vi "Matrix Inverse v1.3.vi"() -> ()   [LabVIEW 2020]
uses:
  <vilib>/Analysis/Matrix/Datatypes/RealMatrix.ctl
  <vilib>/Analysis/baseanly.llb/Mean (DBL).vi
  <vilib>/Analysis/Matrix/Numeric/Conversions/Array To Matrix - RA2.vi
  <vilib>/Analysis/baseanly.llb/Real Inverse Matrix.vi
  <vilib>/Analysis/Matrix/Numeric/Conversions/Matrix To Array - RM.vi
  <vilib>/Analysis/NI_AALBase.lvlib
  <vilib>/Analysis/Matrix/NI_Matrix.lvlib
panel:
  out "pt - pt error":sgl[][](array[numeric])
  out "percent error":dbl format="%0.2f"
  out "x > y?":bool
  out "divide by zero detected":bool
  out "Joint Matrix":sgl[][](array[numeric])
  out "A":T1
  out "sum of error":sgl
  out "inv(A) LABVIEW-FPGA":sgl[][](array[numeric])
  out "inv(A) LABVIEW":T1
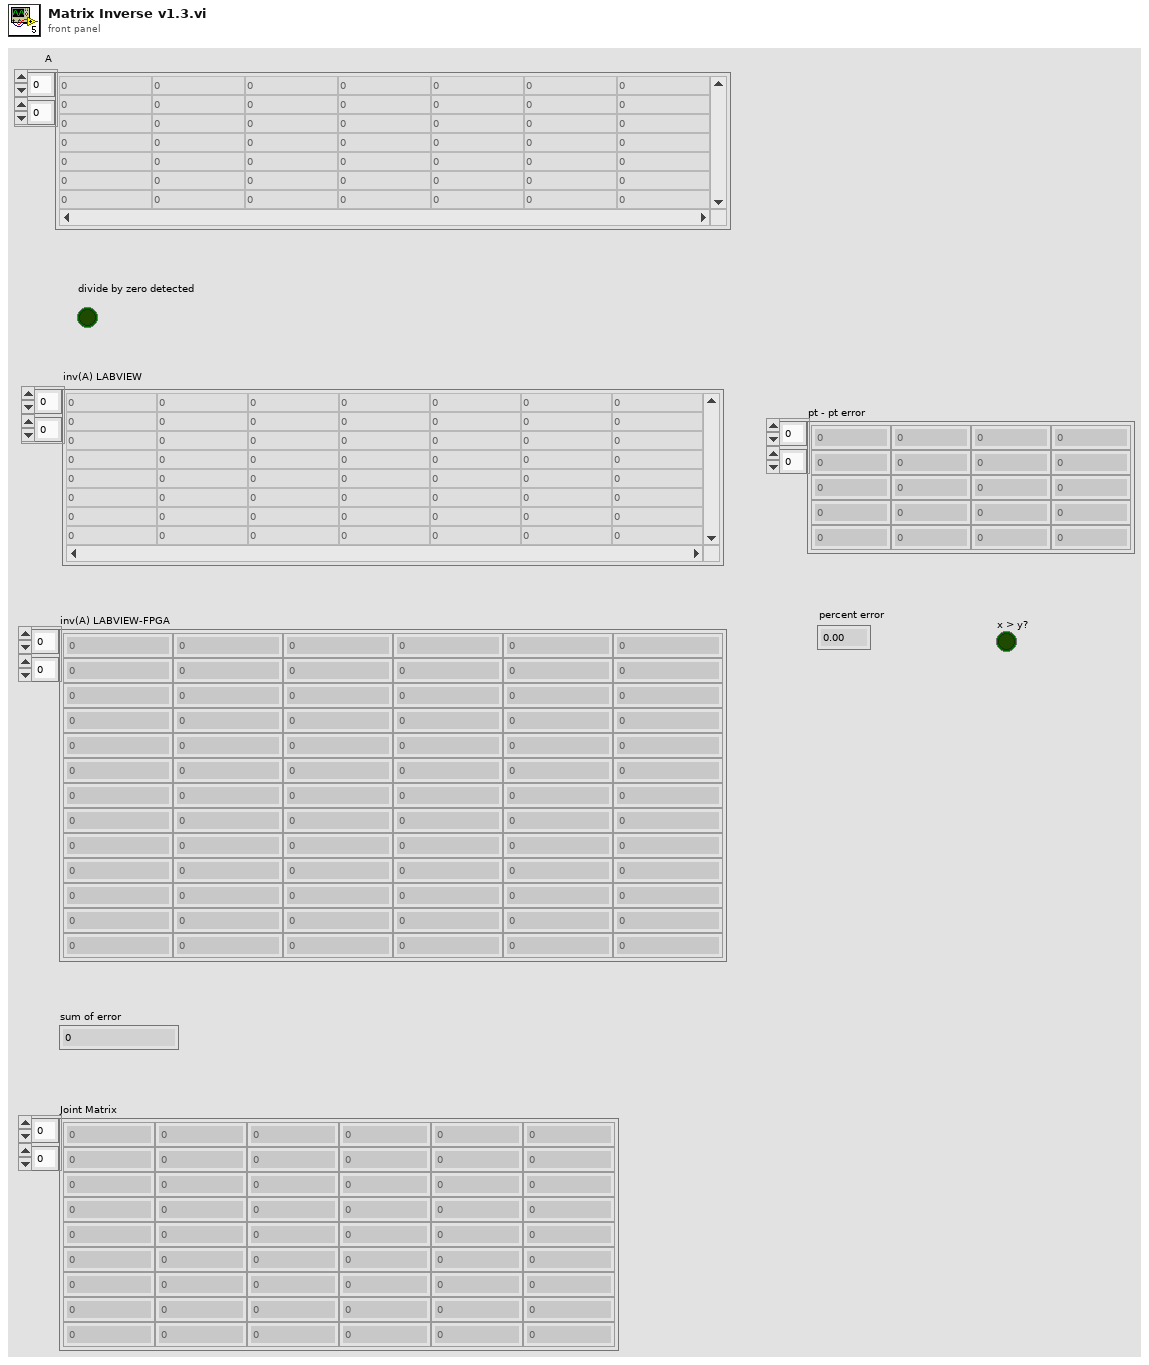
[diagram p1: front panel]
types:
  T1 = typedef "NI_Matrix.lvlib/RealMatrix.ctl" = dbl[][]
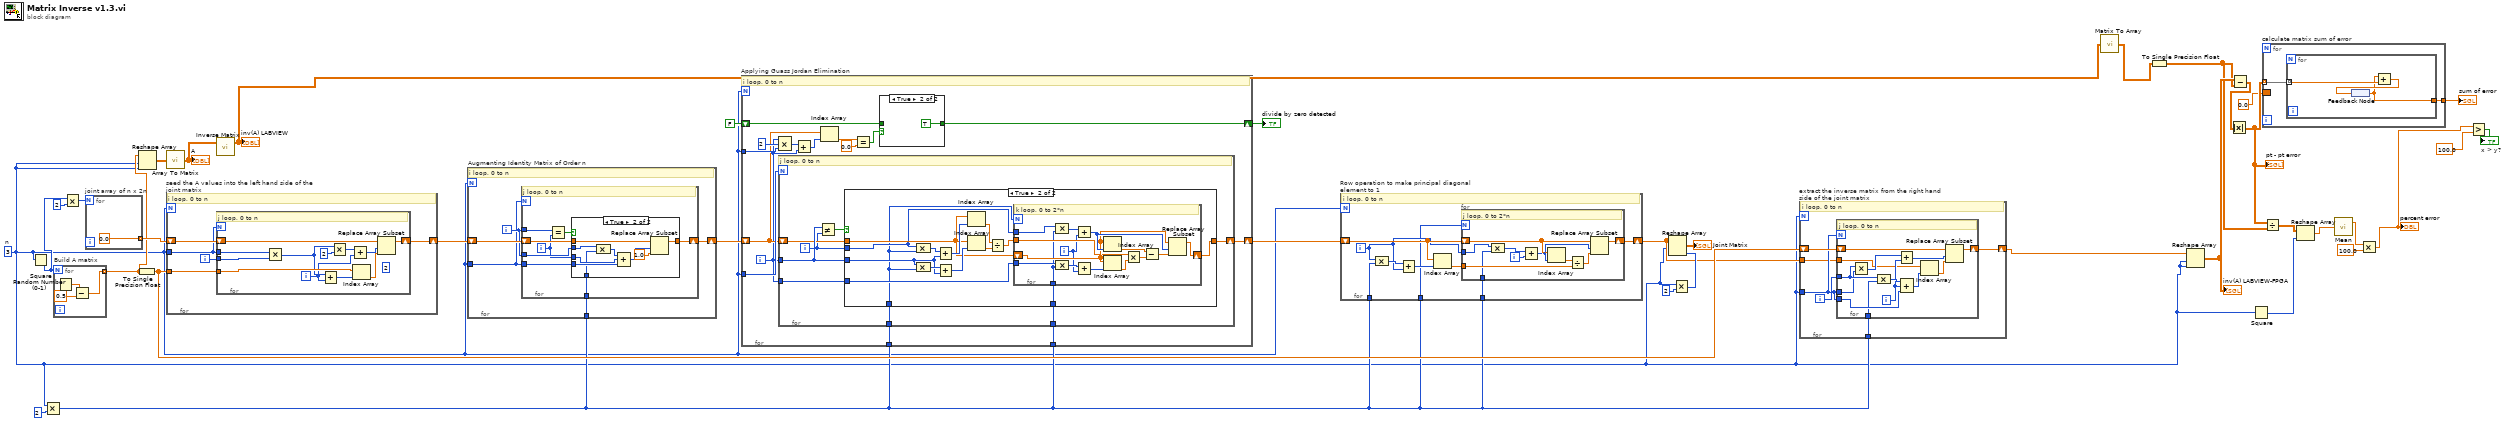
[diagram p0: block diagram]
diagram:
  w4 = 3  # n
  n1 = Square(x=w4) -> (x^2=w17:i32)
  n2 = Multiply(x=w4, y=2) -> (x*y=w15:i32)
  n3 = for "Build A matrix" {
    N: w17 -> [_]
    tunnel: [w38] -> w24 mode=indexing
    n4 = Random Number (0-1)() -> (number: 0 to 1=w40:dbl)
    n5 = Subtract(x=w40, y=0.5) -> (x-y=w38:dbl)
  }
  n6 = Multiply(x=w17, y=2) -> (x*y=w31:i32)
  n7 = for "joint array of n x 2n" {
    N: w31 -> [_]
    tunnel: [sgl 0.0] -> w30 mode=indexing
  }
  n8 = Reshape Array(w24, w4, w4) -> (w37:dbl[][])
  n9 = To Single Precision Float(number=w24) -> (single precision float=w23:sgl[])
  n10 = call-poly <vilib>:"Array To Matrix.vi"("Real 2D Array"=w37) -> ("Real Matrix"=w36:T1)
  "A" <- w36
  n11 = for "seed the A values into the left hand side of the joint matrix" {
    N: w4 -> [_]
    shift-right: [w45] -> w29
    shift-left: w30 -> [w46]
    tunnel: w4 -> [w44]
    tunnel: w23 -> [w43]
    i -> [w42]
    # "i loop, 0 to n"
    n12 = for {
      N: w44 -> [_]
      shift-right: [w57] -> w45
      shift-left: w46 -> [w58]
      tunnel: w44 -> [w54]
      tunnel: w43 -> [w56]
      tunnel: w42 -> [w55]
      i -> [w48]
      (unwired) 2
      # "j loop, 0 to n"
      n13 = Multiply(x=w54, y=w55) -> (x*y=w50:i32)
      n14 = Add(x=w50, y=w48) -> (x+y=w53:i32)
      n15 = Multiply(x=w50, y=2) -> (x*y=w49:i32)
      n16 = Add(x=w49, y=w48) -> (x+y=w47:i32)
      n17 = Index Array(array=w56, index=w53) -> (element=w52:sgl)
      n18 = Replace Array Subset(array=w58, new element=w52, index=w47) -> (w57:sgl[])
    }
  }
  n19 = call-poly <vilib>:"Inverse Matrix.vi"("Input Matrix"=w36) -> ("Inverse Matrix"=w19:T1)  [unwired: 1 in, 1 out]
  "inv(A) LABVIEW" <- w19
  n20 = for "Augmenting Identity Matrix of Order n" {
    N: w4 -> [_]
    shift-right: [w62] -> w26
    shift-left: w29 -> [w63]
    tunnel: w4 -> [w60]
    tunnel: w15 -> [w59]
    i -> [w61]
    # "i loop, 0 to n"
    n21 = for {
      N: w60 -> [_]
      tunnel: w61 -> [w71]
      shift-right: [w68] -> w62
      shift-left: w63 -> [w69]
      tunnel: w61 -> [w67]
      tunnel: w60 -> [w66]
      tunnel: w59 -> [w64]
      i -> [w65]
      # "j loop, 0 to n"
      n22 = Equal?(x=w71, y=w65) -> (x = y?=w70:bool)
      n23 = case shown="True" w70 {
        tunnel: w69 -> [w72 w81]
        tunnel: [w72 w78] -> w68
        tunnel: w67 -> [_ w79]
        tunnel: w66 -> [_ w75]
        tunnel: w65 -> [_ w76]
        tunnel: w64 -> [_ w73]
        frame False {
        }
        frame True {
          n24 = Compound Arithmetic op=MULTIPLY(w79, w73) -> (w77:i32)
          n25 = Compound Arithmetic op=ADD(w77, w76, w75) -> (w74:i32)
          n26 = Replace Array Subset(array=w81, new element=sgl 1.0 ("new element/subarray"), index=w74) -> (w78:sgl[])
        }
      }
    }
  }
  n27 = for "Applying Guass Jordan Elimination" {
    N: w4 -> [_]
    tunnel: w4 -> [w94]
    shift-right: [w88] -> w27
    shift-left: FALSE -> [w89]
    tunnel: w4 -> [w87]
    shift-right: [w84] -> w25
    shift-left: w26 -> [w86]
    tunnel: w15 -> [w83]
    tunnel: w15 -> [w82]
    i -> [w85]
    # "i loop, 0 to n"
    n28 = Compound Arithmetic op=MULTIPLY(w85, 2 ("value"), w94) -> (w93:i32)
    n29 = for {
      N: w87 -> [_]
      tunnel: w85 -> [w104]
      tunnel: w85 -> [w100]
      shift-right: [w99] -> w84
      shift-left: w86 -> [w103]
      tunnel: w83 -> [w98]
      tunnel: w82 -> [w97]
      i -> [w101]
      # "j loop, 0 to n"
      n30 = Not Equal?(x=w104, y=w101) -> (x != y?=w102:bool)
      n31 = case shown="True" w102 {
        tunnel: w104 -> [_ w113]
        tunnel: w103 -> [w105 w112]
        tunnel: w101 -> [_ w111]
        tunnel: w100 -> [_ w109]
        tunnel: [w105 w108] -> w99
        tunnel: w98 -> [_ w107]
        tunnel: w97 -> [_ w106]
        frame False {
        }
        frame True {
          n32 = Compound Arithmetic op=MULTIPLY(w111, w107) -> (w119:i32)
          n33 = Compound Arithmetic op=MULTIPLY(w113, w107) -> (w115:i32)
          n34 = Add(x=w119, y=w113) -> (x+y=w118:i32)
          n35 = Add(x=w115, y=w113) -> (x+y=w114:i32)
          n36 = Index Array(array=w112, index=w118) -> (element=w117:sgl)
          n37 = Index Array(array=w112, index=w114) -> (element=w116:sgl)
          n38 = Divide(x=w117, y=w116) -> (x/y=w110:sgl)
          n39 = for {
            N: w107 -> [_]
            tunnel: w111 -> [w133]
            tunnel: w110 -> [w129]
            tunnel: w109 -> [w126]
            shift-right: [w121] -> w108
            shift-left: w112 -> [w131]
            tunnel: w106 -> [w120]
            i -> [w127]
            # "k loop, 0 to 2*n"
            n40 = Compound Arithmetic op=MULTIPLY(w133, w120) -> (w134:i32)
            n41 = Compound Arithmetic op=MULTIPLY(w126, w120) -> (w128:i32)
            n42 = Add(x=w134, y=w127) -> (x+y=w132:i32)
            n43 = Add(x=w128, y=w127) -> (x+y=w125:i32)
            n44 = Index Array(array=w131, index=w132) -> (element=w123:sgl)
            n45 = Index Array(array=w131, index=w125) -> (element=w130:sgl)
            n46 = Multiply(x=w129, y=w130) -> (x*y=w124:sgl)
            n47 = Subtract(x=w123, y=w124) -> (x-y=w122:sgl)
            n48 = Replace Array Subset(array=w131, new element=w122, index=w132) -> (w121:sgl[])
          }
        }
      }
    }
    n49 = Add(x=w93, y=w85) -> (x+y=w92:i32)
    n50 = Index Array(array=w86, index=w92) -> (element=w91:sgl)
    n51 = Equal?(x=w91, y=sgl 0.0) -> (x = y?=w90:bool)
    n52 = case shown="True" w90 {
      tunnel: w89 -> [w135 _]
      tunnel: [w135 TRUE] -> w88
      frame False {
      }
      frame True {
      }
    }
  }
  "divide by zero detected" <- w27
  n53 = for "Row operation to make principal diagonal element to 1" {
    N: w4 -> [_]
    shift-right: [w140] -> w21
    shift-left: w25 -> [w143]
    tunnel: w15 -> [w139]
    tunnel: w15 -> [w138]
    tunnel: w15 -> [w137]
    i -> [w142]
    # "i loop, 0 to n"
    n54 = Compound Arithmetic op=MULTIPLY(w142, w138) -> (w145:i32)
    n55 = Add(x=w145, y=w142) -> (x+y=w144:i32)
    n56 = Index Array(array=w143, index=w144) -> (element=w141:sgl)
    n57 = for {
      N: w139 -> [_]
      tunnel: w142 -> [w155]
      tunnel: w141 -> [w151]
      shift-right: [w149] -> w140
      shift-left: w143 -> [w150]
      tunnel: w137 -> [w146]
      i -> [w153]
      # "j loop, 0 to 2*n"
      n58 = Compound Arithmetic op=MULTIPLY(w155, w146) -> (w154:i32)
      n59 = Add(x=w154, y=w153) -> (x+y=w148:i32)
      n60 = Index Array(array=w150, index=w148) -> (element=w152:sgl)
      n61 = Divide(x=w152, y=w151) -> (x/y=w147:sgl)
      n62 = Replace Array Subset(array=w150, new element=w147, index=w148) -> (w149:sgl[])
    }
  }
  n63 = Multiply(x=w4, y=2) -> (x*y=w34:i32)
  n64 = Reshape Array(w21, w4, w34) -> (→"Joint Matrix":sgl[][])
  n65 = for "extract the inverse matrix from the right hand side of the joint matrix" {
    N: w4 -> [_]
    tunnel: w4 -> [w158]
    shift-right: [w160] -> w22
    shift-left: w23 -> [w161]
    tunnel: w21 -> [w157]
    tunnel: w15 -> [w156]
    i -> [w159]
    # "i loop, 0 to n"
    n66 = for {
      N: w158 -> [_]
      shift-right: [w173] -> w160
      shift-left: w161 -> [w174]
      tunnel: w159 -> [w170]
      tunnel: w158 -> [w169]
      tunnel: w158 -> [w166]
      tunnel: w157 -> [w164]
      tunnel: w156 -> [w162]
      i -> [w167]
      # "j loop, 0 to n"
      n67 = Multiply(x=w170, y=w169) -> (x*y=w172:i32)
      n68 = Compound Arithmetic op=MULTIPLY(w170, w162) -> (w168:i32)
      n69 = Add(x=w172, y=w167) -> (x+y=w171:i32)
      n70 = Compound Arithmetic op=ADD(w168, w167, w166) -> (w165:i32)
      n71 = Index Array(array=w164, index=w165) -> (element=w163:sgl)
      n72 = Replace Array Subset(array=w174, new element=w163, index=w171) -> (w173:sgl[])
    }
  }
  n73 = call-poly <vilib>:"Matrix To Array.vi"("Real Matrix"=w19) -> ("Real 2D Array"=w18:dbl[][])
  n74 = To Single Precision Float(number=w18) -> (single precision float=w9:sgl[][])
  n75 = Reshape Array(w22, w4, w4) -> (w11:sgl[][])
  "inv(A) LABVIEW-FPGA" <- w11
  n76 = Subtract ("Subtract.vi")(x=w11, y=w9) -> (x-y=w20:sgl[][])
  n77 = Absolute Value ("Absolute Value.vi")(x=w20) -> (abs(x)=w10:sgl[][])
  "pt - pt error" <- w10
  n78 = Square(x=w4) -> (x^2=w3:i32)
  n79 = for "calculate matrix sum of error" {
    tunnel: w10 -> [w176] mode=indexing
    tunnel: [w175] -> w14
    border: sgl 0.0 -> [_]
    n80 = for {
      tunnel: w176 -> [w179] mode=indexing
      tunnel: [w177] -> w175
      n81 = feedback #1() -> (w177:sgl)
      n82 = Add(x=w177, y=w179) -> (x+y=w178:sgl)
      n83 = feedback-in #1(w178) -> ()
    }
  }
  "sum of error" <- w14
  n84 = Divide(x=w10, y=w9) -> (x/y=w8:sgl[][])
  n85 = Reshape Array(w8, w3) -> (w7:sgl[])
  n86 = call-poly <vilib>:"Mean.vi"("X"=w7) -> ("mean"=w6:dbl)  [unwired: 1 out]
  n87 = Multiply(x=w6, y=100.0) -> (x*y=w2:dbl)
  "percent error" <- w2
  n88 = Greater?(x=w2, y=sgl 100.0) -> (0:→"x > y?":bool)
